vi "r cal.vi"(9 "Contact Resistance":dbl, 11 "Array in":dbl[][](array[numeric])) -> (3 "Array out":dbl[][](array[numeric]))   [LabVIEW 2024]
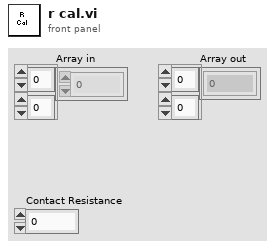
[diagram p1: front panel]
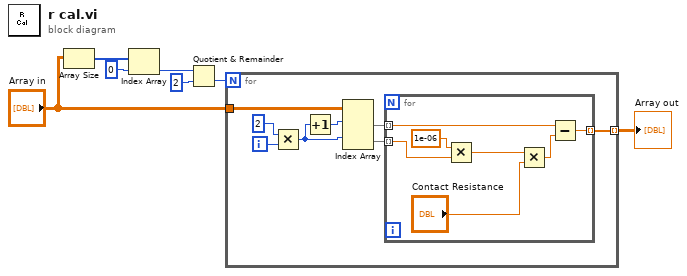
[diagram p0: block diagram]
diagram:
  n1 = Array Size(array="Array in") -> (size(s)=w2:i32[])
  n2 = Index Array(array=w2, index=0) -> (element=w4:i32)
  n3 = Quotient & Remainder(x=w4, y=2) -> (floor(x/y)=w1:i32)  [unwired: 1 out]
  n4 = for {
    N: w1 -> [_]
    tunnel: "Array in" -> [w13]
    tunnel: [w8] -> w7 mode=indexing
    i -> [w15]
    n5 = Multiply(x=2, y=w15) -> (x*y=w11:i32)
    n6 = Increment(x=w11) -> (x+1=w12:i32)
    n7 = Index Array(array=w13, index (row) #1=w12, index (row) #2=w11) -> (element #1=w10:dbl[], element #2=w9:dbl[])  [unwired: 2 in]
    n8 = for {
      tunnel: w10 -> [w19] mode=indexing
      tunnel: w9 -> [w22] mode=indexing
      tunnel: [w17] -> w8 mode=indexing
      n9 = Multiply(x=1e-06, y=w22) -> (x*y=w18:dbl)
      n10 = Multiply(x=w18, y="Contact Resistance") -> (x*y=w21:dbl)
      n11 = Subtract(x=w19, y=w21) -> (x-y=w17:dbl)
    }
  }
  "Array out" <- w7
